vi "ScrollDown.vi"(0 "reference in":refnum<class "DataGridView.lvclass">, 11 "error in (no error)":errorcluster) -> (4 "reference out":refnum<class "DataGridView.lvclass">, 6 "NewRowIndex":i32, 15 "error out":errorcluster)   [LabVIEW 2018, in "DataGridView.lvclass"]
doc: "Scrolls the DataGridView down"
uses:
  DataGridView.lvclass
  System.Windows.Forms
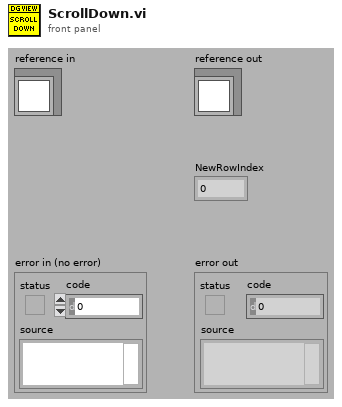
[diagram p1: front panel]
types:
  T1 = typedef "DataGridView.lvclass/ObjectAttributes.ctl" = cluster{"DataGridView":refnum<k24>, "SelectionChangedEvent":refnum<user-event>, "SelectionChanged callback ref":refnum<k27>, "LastSelectedRowIndex":i32}
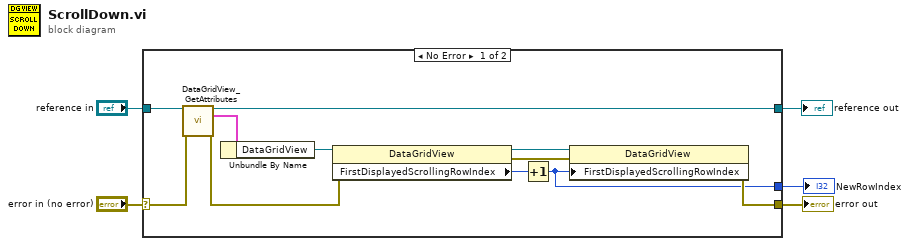
[diagram p0: block diagram]
diagram:
  n1 = case shown="No Error" "error in (no error)" {
    selector: "error in (no error)" -> [w16 w18]
    tunnel: [w7 w18] -> w4
    tunnel: [w13 w17] -> w2
    tunnel: "reference in" -> [w14 w17]
    tunnel: [w6 _] -> w1
    frame No Error {
      n2 = call "DataGridView_GetAttributes.vi"("reference in"=w14, "error in (no error)"=w16) -> ("reference out"=w13:refnum<class "DataGridView.lvclass">, "Data"=w15:T1, "error out"=w8:errorcluster)  [unwired: 10 in, 1 out]
      n3 = Unbundle By Name(w15) -> ("DataGridView"=w9:refnum<k24>)
      n4 = property class="DataGridView"(reference=w9, error in=w8) -> (reference out=w12:refnum<k24>, error out=w10:errorcluster, "FirstDisplayedScrollingRowIndex"=w11:i32)
      n5 = Increment(x=w11) -> (x+1=w6:i32)
      n6 = property class="DataGridView"(reference=w12, error in=w10, "FirstDisplayedScrollingRowIndex"=w6) -> (error out=w7:errorcluster)  [unwired: 1 out]
    }
    frame Error {
    }
  }
  "error out" <- w4
  "reference out" <- w2
  "NewRowIndex" <- w1
